vi "Scale Data.vi"(0 "reference in":refnum<class "Advantech.lvclass">, 1 "Raw Data":dbl, 5 "error in (no error)":errorcluster) -> (14 "reference out":refnum<class "Advantech.lvclass">, 15 "Scaled Data":dbl, 19 "error out":errorcluster)   [LabVIEW 2013, in "Advantech.lvclass"]
uses:
  Advantech.lvclass
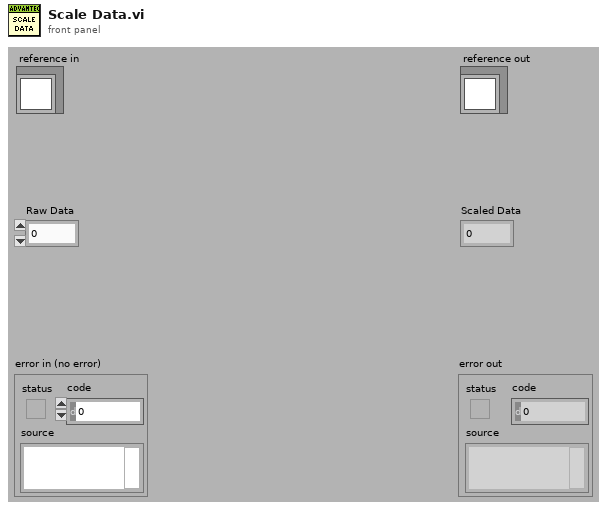
[diagram p1: front panel]
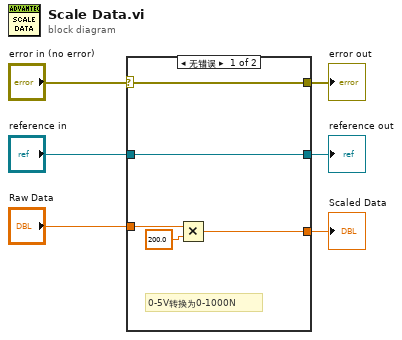
[diagram p0: block diagram]
diagram:
  n1 = case shown="无错误" "error in (no error)" {
    selector: "error in (no error)" -> [w11 w13]
    tunnel: [w11 w13] -> w5
    tunnel: [w7 w12] -> w3
    tunnel: "reference in" -> [w7 w12]
    tunnel: "Raw Data" -> [w10 _]
    tunnel: [w8 _] -> w1
    frame No Error {
      # "0-5V转换为0-1000N"
      n2 = Multiply(x=w10, y=200.0) -> (x*y=w8:dbl)
    }
    frame Error {
    }
  }
  "error out" <- w5
  "reference out" <- w3
  "Scaled Data" <- w1
